vi "保存临时图片.vi"(9 "相机光源":string, 11 "引用句柄输入":T1) -> ()   [LabVIEW 2014]
uses:
  <vilib>/vision/Image Controls.llb/IMAQ Image.ctl
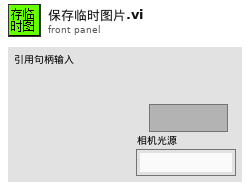
[diagram p1: front panel]
types:
  T1 = typedef "IMAQ Image.ctl" = refnum<image>
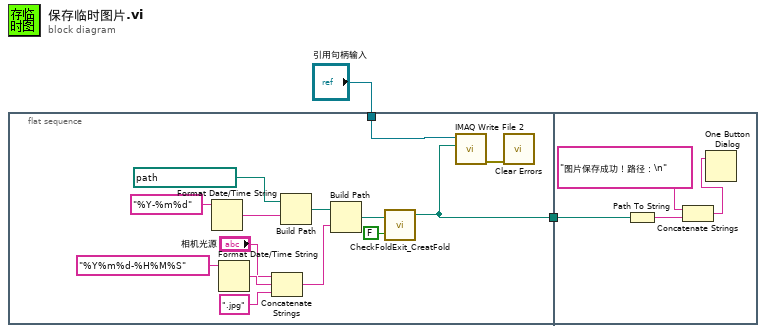
[diagram p0: block diagram]
diagram:
  n1 = flat-sequence {
    tunnel: [w5] -> w2
    tunnel: "引用句柄输入" -> [w4]
    tunnel: w2 -> [w18]
    frame #0 {
      n2 = Format Date/Time String(time format string (%c)="%Y-%m%d") -> (date/time string=w12:string)  [unwired: 2 in]
      n3 = Format Date/Time String(time format string (%c)="%Y%m%d-%H%M%S") -> (date/time string=w11:string)  [unwired: 2 in]
      n4 = Concatenate Strings("相机光源", w11, ".jpg" ("string")) -> (w8:string)
      n5 = Build Path(base path=path "D:/临时存档图片" ("File Path"), name or relative path=w12) -> (appended path=w9:path)
      n6 = Build Path(base path=w9, name or relative path=w8) -> (appended path=w6:path)
      n7 = call "CheckFoldExit_CreatFold.vi"("path in"=w6, "FoldOrFile¡H"=FALSE) -> ("File out"=w5:path)  [unwired: 2 out]
      n8 = call-poly "IMAQ Write File 2"("File Path"=w5, "Image"=w4) -> ("error out"=w16:errorcluster)  [unwired: 8 in, 1 out]
      n9 = call <vilib>:"Clear Errors.vi"("error in (no error)"=w16) -> ()  [unwired: 5 in, 2 out]
    }
    frame #1 {
      n10 = Path To String(path=w18) -> (string=w19:string)
      n11 = Concatenate Strings("图片保存成功！路径：\n" ("消息"), w19) -> (w17:string)
      n12 = One Button Dialog(message=w17) -> ()  [unwired: 1 in, 1 out]
    }
  }
